vi "MessungNeukurve.vi"(0 "Spannungs Abweichung":dbl=5.0, 1 "maximale Spannung":dbl=10.0, 2 "Frequency (1000 Hz)":dbl=1000.0, 3 "Messpunkte Oszi (6000)":i32=6000, 5 "VISA Name OZ In (OZ)":refnum<visa-resource-name>="USB0::0x0957::0x179B::MY54313507::INSTR", 6 "VISA Name FG in":refnum<visa-resource-name>="USB0::0x0957::0x0407::MY44043889::INSTR", 7 "error in":errorcluster, 8 "faktor2":dbl, 10 "Faktor Runge Kutta":dbl=700.0, 12 "Anzahl Messpunkte Neukurve":i8=16 min=10 max=30 step=1) -> (20 "HB Matrix":T1, 21 "Output B Array":dbl[](array[numeric]), 22 "Output H Array":dbl[](array[numeric]), 25 "VISA Name OZ Out":refnum<visa-resource-name>="USB0::0x0957::0x179B::MY54313507::INSTR", 26 "VISA Name FG out":refnum<visa-resource-name>, 27 "error out":errorcluster)   [LabVIEW 2016]
uses:
  <vilib>/Analysis/Matrix/Datatypes/RealMatrix.ctl
  controls/Oszi_KanalInfo.ctl
  <instrlib>/Agilent 33XXX Series/Agilent 33XXX Series.lvlib
  <vilib>/Analysis/Matrix/NI_Matrix.lvlib
panel:
  out "Waveform Chart":u32(graph)
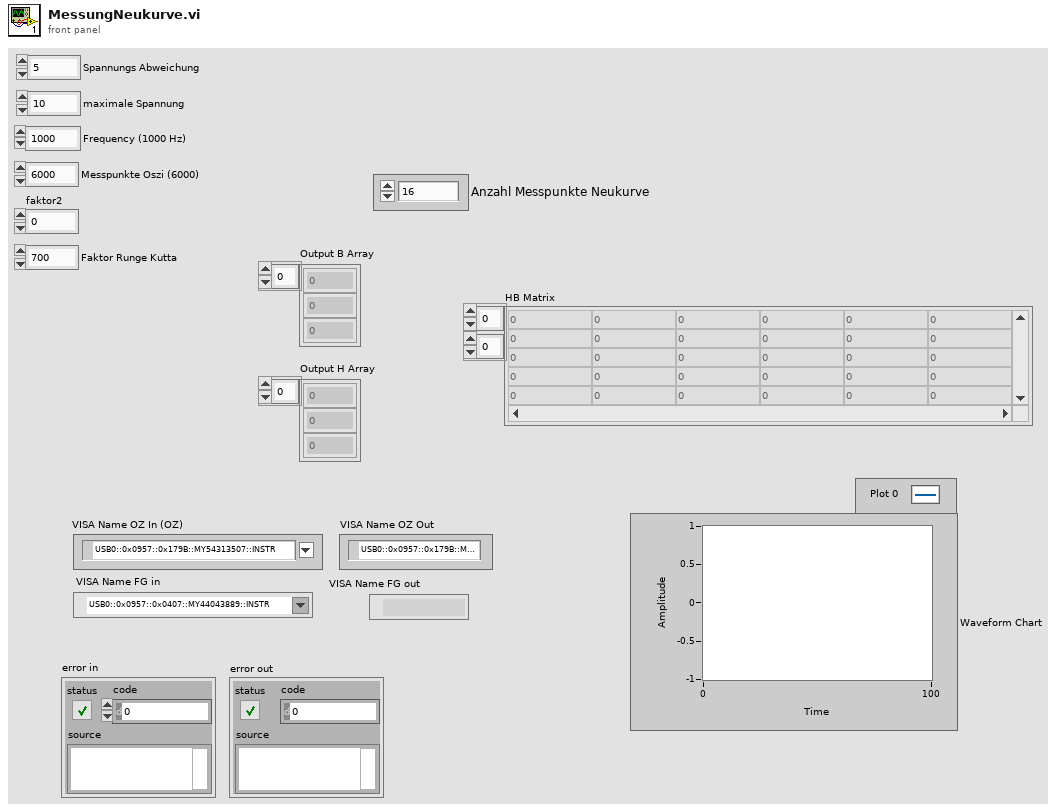
[diagram p1: front panel]
types:
  T1 = typedef "NI_Matrix.lvlib/RealMatrix.ctl" = dbl[][]
  T2 = typedef "Oszi_KanalInfo.ctl" = dbl
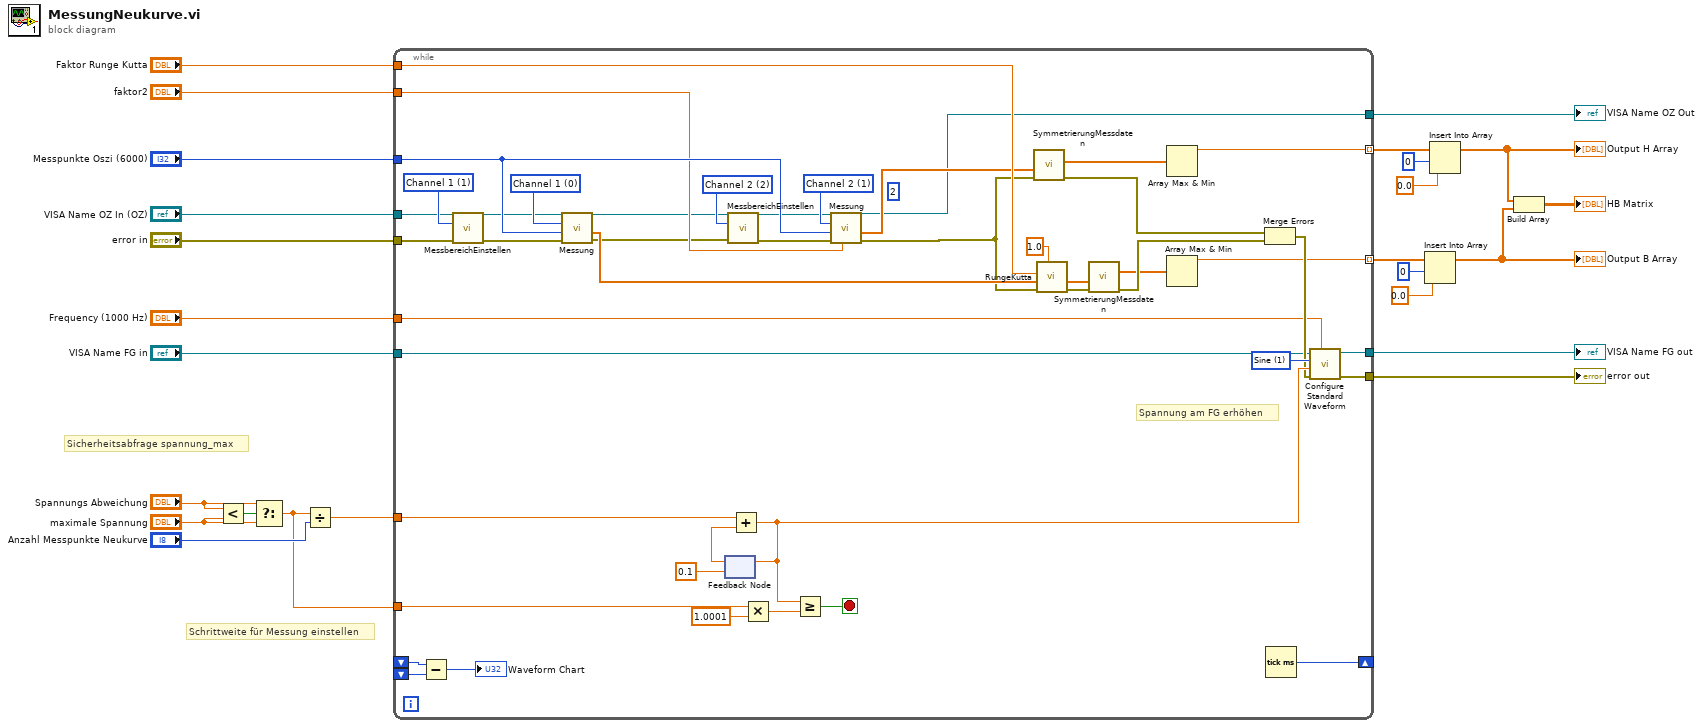
[diagram p0: block diagram]
diagram:
  # "Sicherheitsabfrage spannung_max"
  # "Schrittweite für Messung einstellen"
  n1 = Less?(x="Spannungs Abweichung", y="maximale Spannung") -> (x < y?=w25:bool)
  n2 = Select(t="Spannungs Abweichung", s=w25, f="maximale Spannung") -> (s? t:f=w1:dbl)
  n3 = Divide(x=w1, y="Anzahl Messpunkte Neukurve") -> (x/y=w2:dbl)
  n4 = while {
    tunnel: w2 -> [w66]
    tunnel: w1 -> [w65]
    tunnel: "error in" -> [w50]
    tunnel: "VISA Name FG in" -> [w35]
    tunnel: [w62] -> w22
    tunnel: [w59] -> w21
    tunnel: [w52] -> w4 mode=indexing
    tunnel: [w28] -> w10 mode=indexing
    tunnel: "VISA Name OZ In (OZ)" -> [w48]
    tunnel: "Faktor Runge Kutta" -> [w61]
    tunnel: [w29] -> w20
    tunnel: "Frequency (1000 Hz)" -> [w43]
    tunnel: "faktor2" -> [w36]
    tunnel: "Messpunkte Oszi (6000)" -> [w56]
    shift-right: [w41] -> _
    shift-left: _ -> [w39]
    shift-left: _ -> [w40]
    stop <- w69 stop-if-true
    (unwired) 2 ("Channel")
    w55 = 0 items=["Channel 1"=0, "Channel 2"=1, "Channel 3"=2, "Channel 4"=3, "Waveform Memory 1"=5, "Waveform Memory 2"=6, "Serial Bus 1"=7, "Serial Bus 2"=8, "Digital Bus Low"=9, "Digital Bus High "=10, "Digital Bus 1"=11, "Digital Bus 2"=12, "Function 1"=32, "Function 2"=33, "Function 3"=34, "Function 4"=35, "Math 1"=36, "Math 2"=37, "Math 3"=38, "Math 4"=39] ("Source Channel (0: Channel 1)")
    w57 = 1 items=["Channel 1"=0, "Channel 2"=1, "Channel 3"=2, "Channel 4"=3, "Waveform Memory 1"=5, "Waveform Memory 2"=6, "Serial Bus 1"=7, "Serial Bus 2"=8, "Digital Bus Low"=9, "Digital Bus High "=10, "Digital Bus 1"=11, "Digital Bus 2"=12, "Function 1"=32, "Function 2"=33, "Function 3"=34, "Function 4"=35, "Math 1"=36, "Math 2"=37, "Math 3"=38, "Math 4"=39] ("Source Channel (0: Channel 1)")
    w49 = 1 items=["Channel 1"=1, "Channel 2"=2, "Channel 3"=3, "Channel 4"=4] ("Channel Name (1: Channel 1)")
    w45 = 2 items=["Channel 1"=1, "Channel 2"=2, "Channel 3"=3, "Channel 4"=4] ("Channel Name (1: Channel 1)")
    w64 = u16 1 items=["DC", "Sine", "Square", "Triangle", "Ramp", "Pulse", "Noise", "Sinc", "Negative Ramp", "Exponential Rise", "Exponential Fall", "Cardiac"] ("Waveform Function (1: Sine)")
    # "Spannung am FG erhöhen"
    n5 = Subtract(x=w39, y=w40) -> (x-y=→"Waveform Chart":u32)
    n6 = call "MessbereichEinstellen.vi"("Error_in"=w50, "Channel Name (1: Channel 1)"=w49, "VISA Name OZ in(OZ)"=w48) -> ("Error_out"=w51:errorcluster, "VISA Name OZ out"=w47:refnum<visa-resource-name>)  [unwired: 7 in]
    n7 = call "Messung.vi"("error in"=w51, "Points"=w56, "Source Channel (0: Channel 1)"=w55, "VISA resource name"=w47) -> ("error out"=w32:errorcluster, "Messdaten"=w33:dbl[], "VISA resource name out"=w31:refnum<visa-resource-name>)  [unwired: 4 in, 1 out]
    n8 = feedback #1(0.1) -> (w70:dbl)
    n9 = call "MessbereichEinstellen.vi"("Error_in"=w32, "Channel Name (1: Channel 1)"=w45, "VISA Name OZ in(OZ)"=w31) -> ("Error_out"=w46:errorcluster, "VISA Name OZ out"=w44:refnum<visa-resource-name>)  [unwired: 7 in]
    n10 = Add(x=w66, y=w70) -> (x+y=w63:dbl)
    n11 = feedback-in #1(w63) -> ()
    n12 = Multiply(x=w65, y=1.0001) -> (x*y=w68:dbl)
    n13 = Greater Or Equal?(x=w63, y=w68) -> (x >= y?=w69:bool)
    n14 = call "Messung.vi"("Faktor2 (1)"=w36, "error in"=w46, "Points"=w56, "Source Channel (0: Channel 1)"=w57, "VISA resource name"=w44) -> ("error out"=w30:errorcluster, "Messdaten"=w37:dbl[], "VISA resource name out"=w29:refnum<visa-resource-name>)  [unwired: 3 in, 1 out]
    n15 = call "SymmetrierungMessdaten.vi"("error in"=w30, "Input Array"=w37) -> ("error out"=w34:errorcluster, "Output Array"=w54:dbl[])  [unwired: 3 in, 3 out]
    n16 = call "RungeKutta.vi"("Oszi-Channel (1)"=T2 1.0, "error in (no error)"=w30, "Messdaten In"=w33, "faktor1"=w61) -> ("error out"=w27:errorcluster, "Output Array"=w26:dbl[])  [unwired: 6 in]
    n17 = call "SymmetrierungMessdaten.vi"("error in"=w27, "Input Array"=w26) -> ("error out"=w58:errorcluster, "Output Array"=w53:dbl[])  [unwired: 3 in, 3 out]
    n18 = Array Max & Min(array=w54) -> (max value=w28:dbl)  [unwired: 3 out]
    n19 = Array Max & Min(array=w53) -> (max value=w52:dbl)  [unwired: 3 out]
    n20 = Merge Errors(w34, w58) -> (w60:errorcluster)
    n21 = Tick Count (ms)() -> (millisecond timer value=w41:u32)
    n22 = call <instrlib>:"Configure Standard Waveform.vi"("Frequency (1000 Hz)"=w43, "error in (no error)"=w60, "Amplitude (1)"=w63, "Waveform Function (1: Sine)"=w64, "VISA resource name"=w35) -> ("error out"=w59:errorcluster, "VISA resource name out"=w62:refnum<visa-resource-name>)  [unwired: 5 in]
  }
  "error out" <- w21
  "VISA Name FG out" <- w22
  "VISA Name OZ Out" <- w20
  n23 = Insert Into Array(array=w4, index=0 ("Index"), new element=0.0 ("Neues Element/Teil-Array")) -> (w5:dbl[])
  "Output B Array" <- w5
  n24 = Insert Into Array(array=w10, index=0 ("Index"), new element=0.0 ("Neues Element/Teil-Array")) -> (w8:dbl[])
  "Output H Array" <- w8
  n25 = Build Array(w8, w5) -> (→"HB Matrix":T1)
